vi "MCL Get Clock Frequency.vi"(8 "error in (no error)":errorcluster, 9 "handle":i32, 10 "dacfreq":dbl, 11 "adcfreq":dbl) -> (0 "error out":errorcluster, 1 "function return":i32, 2 "dacfreq out":dbl, 3 "adcfreq out":dbl)   [LabVIEW 2014, in "Madlib.lvlib"]
doc: "MADLIB_API int MCL_GetClockFrequency(double *adcfreq, double *dacfreq, int handle);"
uses:
  <userlib>/Lambda2/lib/Madlib/Madlib.lvlib
  <userlib>/Lambda2/lib/Madlib/Madlib.dll
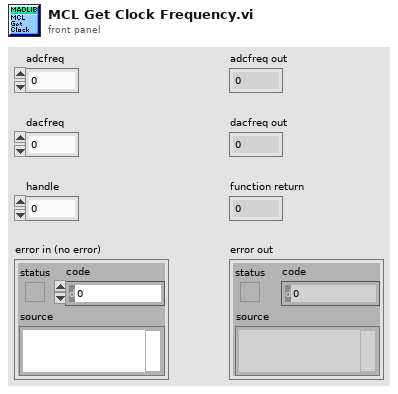
[diagram p1: front panel]
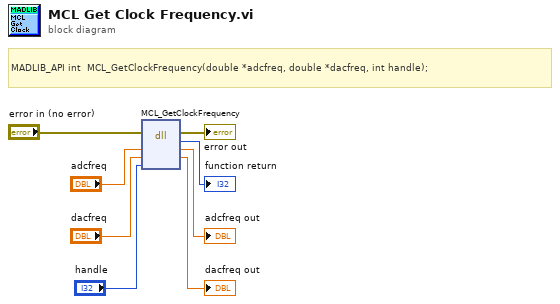
[diagram p0: block diagram]
diagram:
  # "MADLIB_API\tint\t\tMCL_GetClockFrequency(double *adcfreq, double *dacfreq, int handle);"
  n1 = dll-call lib="C:/Program Files (x86)/National Instruments/LabVIEW 2014/user.lib/Lambda2/lib/Madlib/Madlib.*" fn="MCL_GetClockFrequency"(error in="error in (no error)", "adcfreq"="adcfreq", "dacfreq"="dacfreq", "handle"="handle") -> (error out=→"error out":errorcluster, →"function return":i32, "adcfreq"=→"adcfreq out":dbl, "dacfreq"=→"dacfreq out":dbl)  [unwired: 3 in, 1 out]
